vi "Set Smart GFI.vi"(8 "error IO":errorcluster, 9 "Smart GFI":dbl, 11 "VISA resource name":refnum<visa-resource-name>) -> (0 "error Out":errorcluster, 3 "VISA resource Out":refnum<visa-resource-name>)   [LabVIEW 2012, in "Associated Research 78XX Series.lvlib"]
uses:
  <instrlib>/Associated Research 78XX Series/Associated Research 78XX Series.lvlib
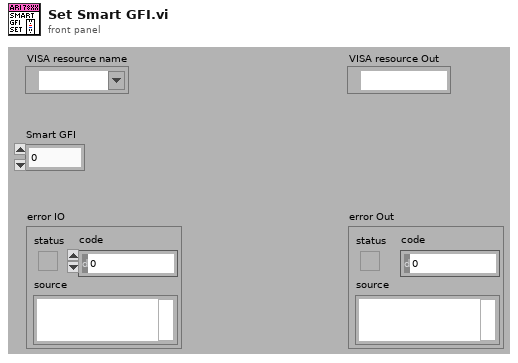
[diagram p1: front panel]
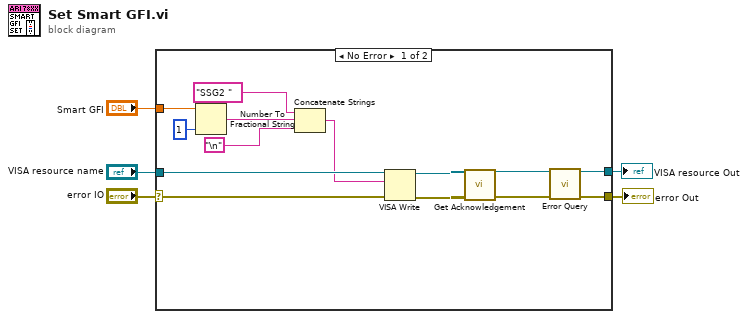
[diagram p0: block diagram]
diagram:
  n1 = case shown="No Error" "error IO" {
    selector: "error IO" -> [w19 w21]
    tunnel: [w16 w21] -> w2
    tunnel: [w17 w20] -> w3
    tunnel: "VISA resource name" -> [w18 w20]
    tunnel: "Smart GFI" -> [w10 _]
    frame No Error {
      n2 = Number To Fractional String(number=w10, precision (6)=i16 1) -> (F-format string=w9:string)  [unwired: 2 in]
      n3 = Concatenate Strings("SSG2 " ("Command to Send (empty)"), w9, "\n") -> (w13:string)
      n4 = VISA Write(VISA resource name=w18, write buffer=w13, error in (no error)=w19) -> (VISA resource name out=w7:refnum<visa-resource-name>, error out=w6:errorcluster)  [unwired: 1 out]
      n5 = call <instrlib>:"Get Acknowledgement.vi"("VISA resource name"=w7, "error in (no error)"=w6) -> ("VISA resource name out"=w12:refnum<visa-resource-name>, "error out"=w11:errorcluster)  [unwired: 12 in]
      n6 = call <instrlib>:"Error Query.vi"("VISA resource name"=w12, "error in (no error)"=w11) -> ("VISA resource name out"=w17:refnum<visa-resource-name>, "error out"=w16:errorcluster)  [unwired: 10 in, 2 out]
    }
    frame Error {
    }
  }
  "VISA resource Out" <- w3
  "error Out" <- w2
